vi "ITC 503 -- PID table to pid.vi"(9 "temperature":dbl, 10 "PID table":dbl[][](array[numeric])=[[400.0, 10.0, 3.0, 1.0], [300.0, 10.0, 3.0, 1.0], [60.0, 10.0, 3.0, 1.0], [40.0, 10.0, 3.0, 1.0], [20.0, 30.0, 0.5, 0.2], [10.0, 40.0, 0.5, 0.2], [1.0, 50.0, 0.2, 0.2], [0.0, 50.0, 0.2, 0.2]]) -> (0 "D":dbl, 1 "I":dbl, 2 "P":dbl)   [LabVIEW 2012]
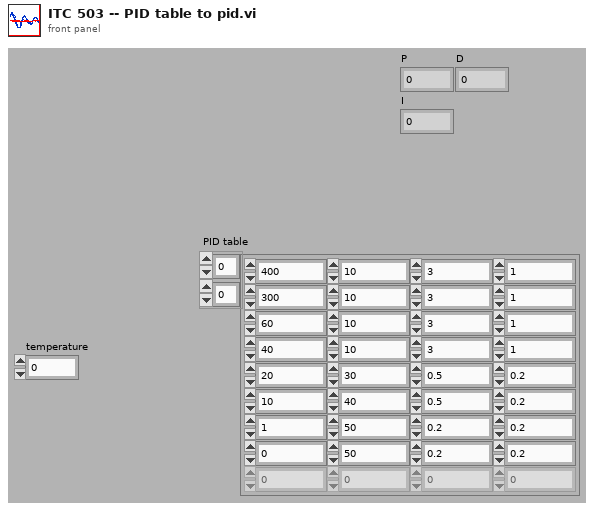
[diagram p1: front panel]
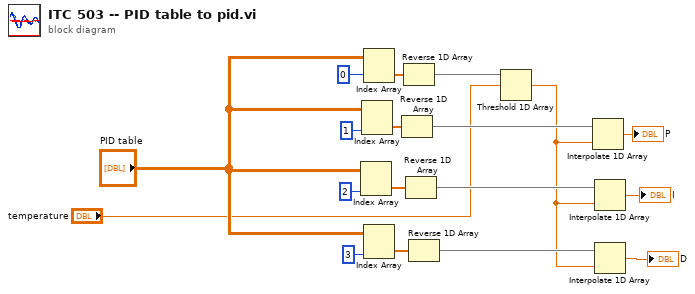
[diagram p0: block diagram]
diagram:
  n1 = Index Array(array="PID table", index (col)=2 ("disabled index (col)")) -> (element=w16:dbl[])  [unwired: 1 in]
  n2 = Index Array(array="PID table", index (col)=1 ("disabled index (col)")) -> (element=w17:dbl[])  [unwired: 1 in]
  n3 = Index Array(array="PID table", index (col)=0 ("disabled index (col)")) -> (element=w11:dbl[])  [unwired: 1 in]
  n4 = Index Array(array="PID table", index (col)=3 ("disabled index (col)")) -> (element=w13:dbl[])  [unwired: 1 in]
  n5 = Reverse 1D Array(array=w17) -> (reversed array=w18:dbl[])
  n6 = Reverse 1D Array(array=w11) -> (reversed array=w12:dbl[])
  n7 = Reverse 1D Array(array=w16) -> (reversed array=w15:dbl[])
  n8 = Reverse 1D Array(array=w13) -> (reversed array=w14:dbl[])
  n9 = Threshold 1D Array(2:"temperature", 3:w12) -> (0:w10:dbl)  [unwired: 1 in]
  n10 = Interpolate 1D Array(1:w10, 2:w18) -> (0:→"P":dbl)
  n11 = Interpolate 1D Array(1:w10, 2:w15) -> (0:→"I":dbl)
  n12 = Interpolate 1D Array(1:w10, 2:w14) -> (0:→"D":dbl)
